vi "Write Values and Check for Stabilization.vi"(0 "DataCluster In":T1, 5 "DesiredParameters":T3={"Para1"=0, "SP1"=0.0, "Para2"=1, "SP2"=0.0, "Para3"=4, "SP3"=10.0}, 7 "Stability Cluster":T2, 9 "Controller?":bool, 11 "DataDisplayRefs":refnum<vi>[](array[refnum]), 13 "StabilizedRef":refnum<vi>) -> (4 "DataCluster Out":T1)   [LabVIEW 2019]
uses:
  TypeDef/DataCluster.ctl
  TypeDef/Command Cluster.ctl
  TypeDef/Stability Cluster.ctl
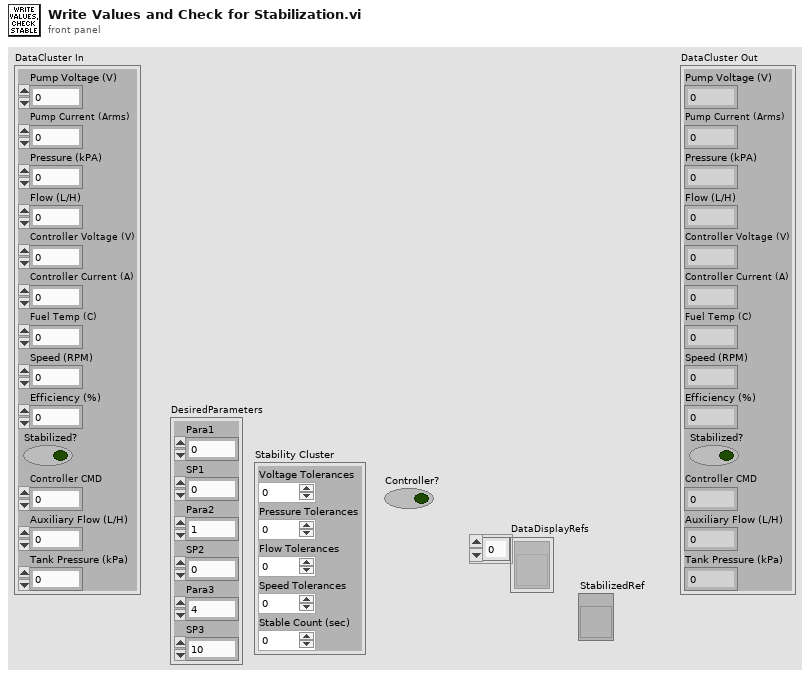
[diagram p1: front panel]
types:
  T1 = typedef "DataCluster.ctl" = cluster{"Pump Voltage (V)":dbl, "Pump Current (Arms)":dbl, "Pressure (kPA)":dbl, "Flow (L/H)":dbl, "Controller Voltage (V)":dbl, "Controller Current (A)":dbl, "Fuel Temp (C)":dbl, "Speed (RPM)":dbl, "Efficiency (%)":dbl, "Stabilized?":bool, "Controller CMD":dbl, "Auxiliary Flow (L/H)":dbl, "Tank Pressure (kPa)":dbl}
  T2 = typedef "Stability Cluster.ctl" = cluster{"Voltage Tolerances":dbl, "Pressure Tolerances":dbl, "Flow Tolerances":dbl, "Speed Tolerances":dbl, "Stable Count (sec)":dbl}
  T3 = typedef "Command Cluster.ctl" = cluster{"Para1":i32, "SP1":dbl, "Para2":i32, "SP2":dbl, "Para3":i32, "SP3":dbl}
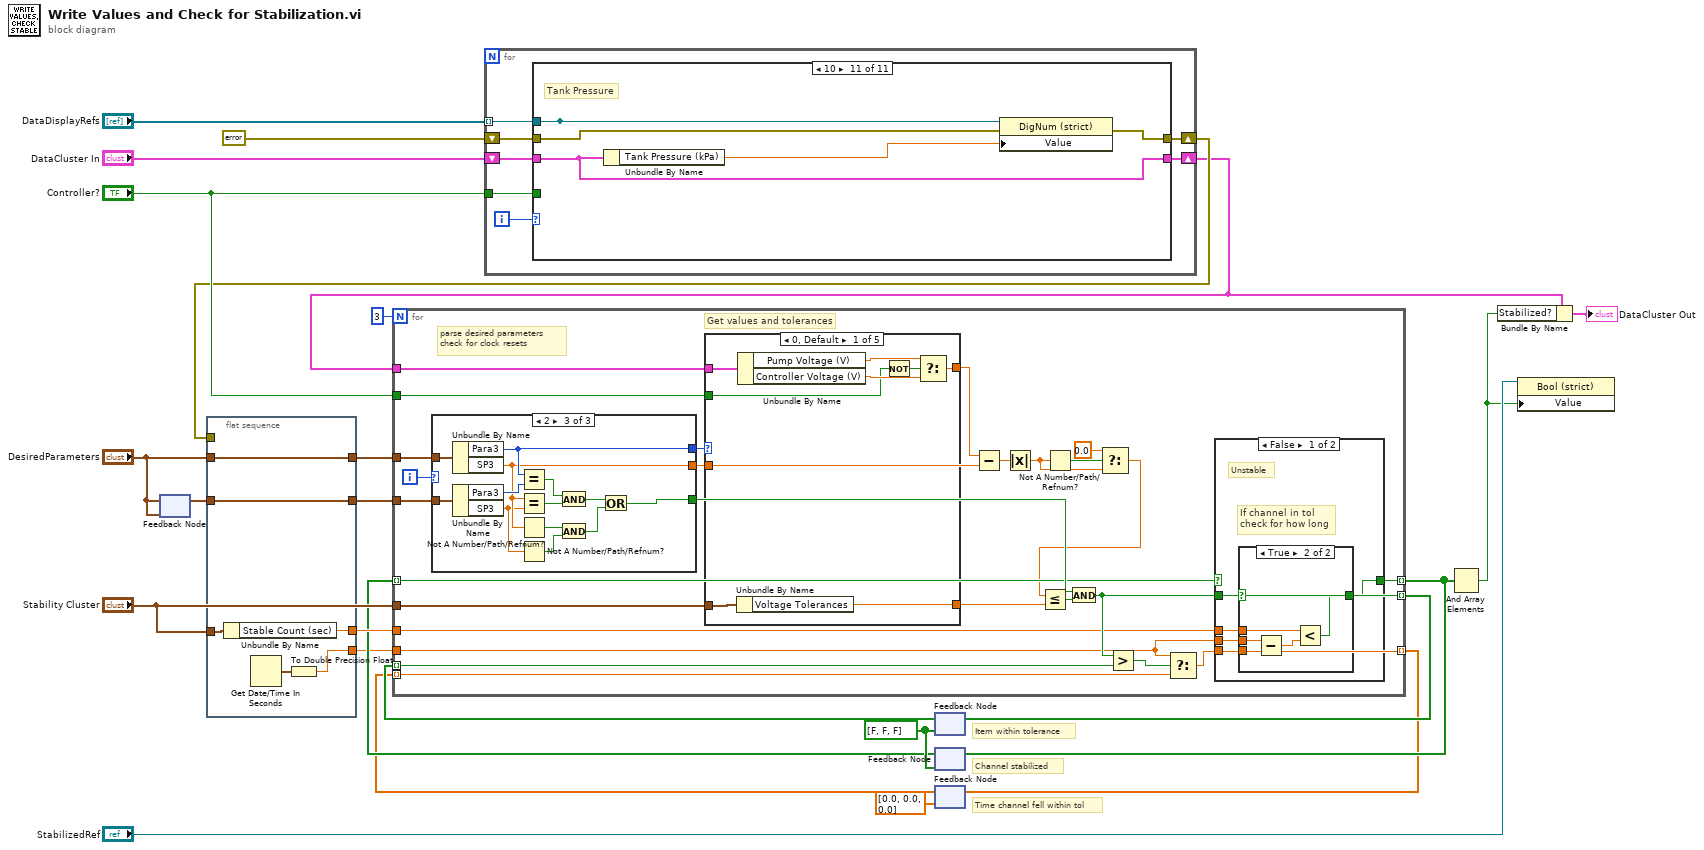
[diagram p0: block diagram]
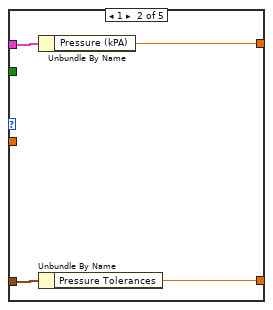
[diagram p4: hidden frame]
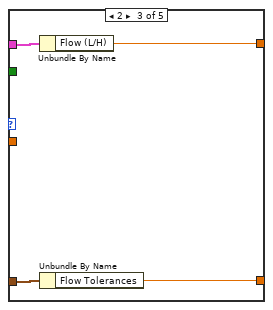
[diagram p5: hidden frame]
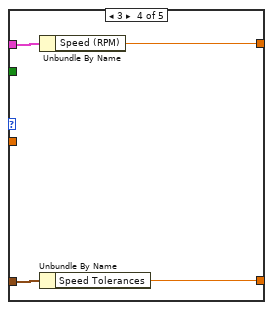
[diagram p6: hidden frame]
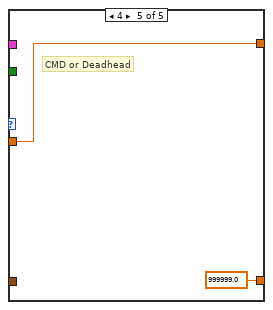
[diagram p7: hidden frame]
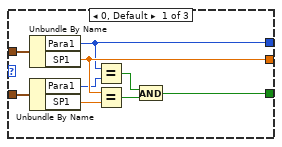
[diagram p8: hidden frame]
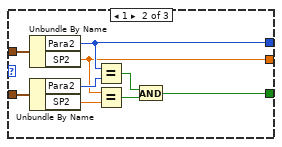
[diagram p9: hidden frame]
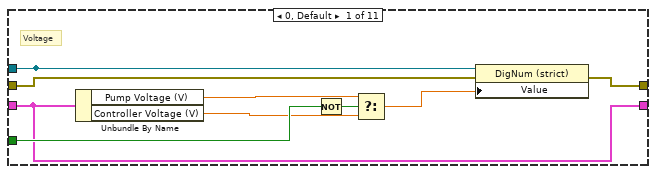
[diagram p10: hidden frame]
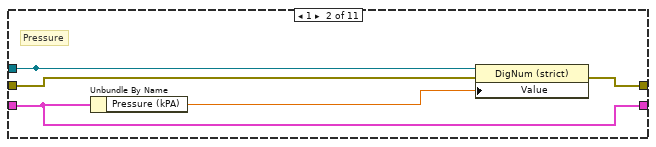
[diagram p11: hidden frame]
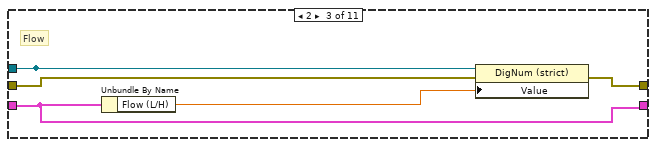
[diagram p12: hidden frame]
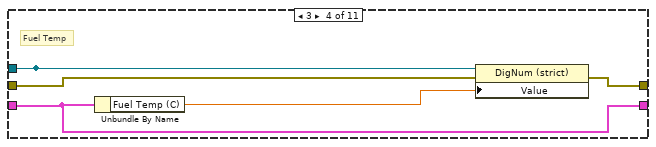
[diagram p13: hidden frame]
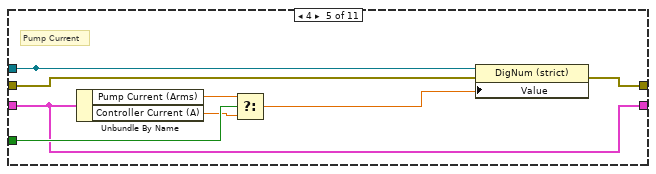
[diagram p14: hidden frame]
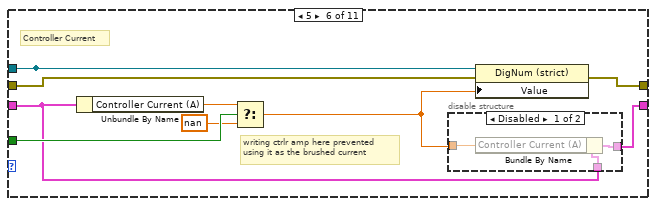
[diagram p15: hidden frame]
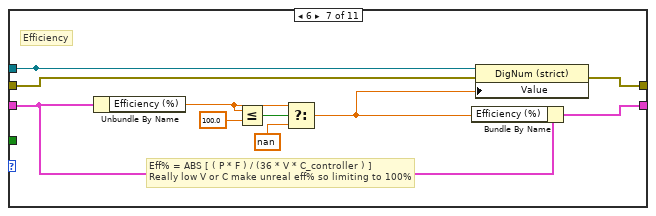
[diagram p17: hidden frame]
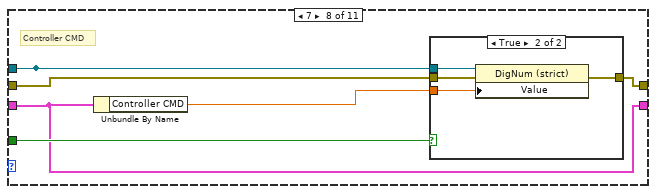
[diagram p18: hidden frame]
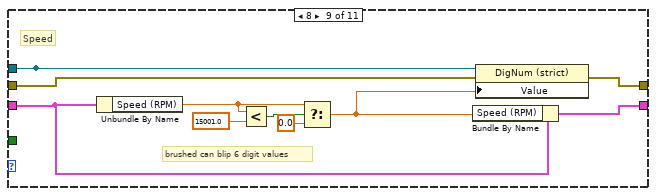
[diagram p20: hidden frame]
diagram:
  w18 = bool[] [FALSE, FALSE, FALSE]
  # "Time channel fell within tol"
  # "Channel stabilized"
  # "Item within tolerance"
  n1 = feedback-in #1("DesiredParameters") -> ()
  n2 = feedback #1("DesiredParameters") -> (w7:T3)
  n3 = flat-sequence {
    tunnel: "Stability Cluster" -> [w31]
    tunnel: [w30] -> w21
    tunnel: "DesiredParameters" -> [w29]
    tunnel: w7 -> [w28]
    tunnel: [w29] -> w6
    tunnel: [w28] -> w5
    tunnel: [w26] -> w4
    tunnel: w3 -> [_]
    frame #0 {
      n4 = Unbundle By Name(w31) -> ("Stable Count (sec)"=w30:dbl)
      n5 = Get Date/Time In Seconds() -> (seconds since 1Jan1904=w27:timestamp)
      n6 = To Double Precision Float(number=w27) -> (double precision float=w26:dbl)
    }
  }
  n7 = for {
    tunnel: "Controller?" -> [w36]
    tunnel: "DataDisplayRefs" -> [w35] mode=indexing
    shift-right: [w33] -> w3
    shift-left: errorcluster {"status"=FALSE, "code"=0, "source"=""} ("error in (no error)") -> [w34]
    shift-right: [w32] -> w1
    shift-left: "DataCluster In" -> [w37]
    i -> [w38]
    n8 = case shown="10" w38 {
      tunnel: w37 -> [w39 w48 w53 w58 w63 w73 w86 w94 w107 w115 w120]
      tunnel: w36 -> [w46 _ _ _ w67 w77 _ w97 _ _ _]
      tunnel: [w43 w52 w57 w62 w70 w79 w93 w99 w114 w119 w124] -> _
      tunnel: w35 -> [w43 w52 w57 w62 w70 w79 w93 w99 w114 w119 w124]
      tunnel: w34 -> [w41 w49 w55 w60 w65 w75 w88 w96 w109 w118 w123]
      tunnel: [w40 w50 w54 w59 w64 w74 w87 w95 w108 w117 w122] -> w33
      tunnel: [w39 w48 w53 w58 w63 w71 w85 w94 w105 w115 w120] -> w32
      frame 0, Default {
        # "Voltage"
        n9 = Unbundle By Name(w39) -> ("Pump Voltage (V)"=w45:dbl, "Controller Voltage (V)"=w44:dbl)
        n10 = Not(x=w46) -> (.not. x?=w47:bool)
        n11 = Select(t=w45, s=w47, f=w44) -> (s? t:f=w42:dbl)
        n12 = property class="DigNum (strict)"(reference=w43, error in=w41, "Value"=w42) -> (error out=w40:errorcluster)  [unwired: 1 out]
      }
      frame 1 {
        # "Pressure"
        n13 = Unbundle By Name(w48) -> ("Pressure (kPA)"=w51:dbl)
        n14 = property class="DigNum (strict)"(reference=w52, error in=w49, "Value"=w51) -> (error out=w50:errorcluster)  [unwired: 1 out]
      }
      frame 2 {
        # "Flow"
        n15 = Unbundle By Name(w53) -> ("Flow (L/H)"=w56:dbl)
        n16 = property class="DigNum (strict)"(reference=w57, error in=w55, "Value"=w56) -> (error out=w54:errorcluster)  [unwired: 1 out]
      }
      frame 3 {
        # "Fuel Temp"
        n17 = Unbundle By Name(w58) -> ("Fuel Temp (C)"=w61:dbl)
        n18 = property class="DigNum (strict)"(reference=w62, error in=w60, "Value"=w61) -> (error out=w59:errorcluster)  [unwired: 1 out]
      }
      frame 4 {
        # "Pump Current"
        n19 = Unbundle By Name(w63) -> ("Pump Current (Arms)"=w69:dbl, "Controller Current (A)"=w66:dbl)
        n20 = Select(t=w69, s=w67, f=w66) -> (s? t:f=w68:dbl)
        n21 = property class="DigNum (strict)"(reference=w70, error in=w65, "Value"=w68) -> (error out=w64:errorcluster)  [unwired: 1 out]
      }
      frame 5 {
        # "writing ctrlr amp here prevented\nusing it as the brushed current"
        # "Controller Current"
        n22 = Unbundle By Name(w73) -> ("Controller Current (A)"=w78:dbl)
        n23 = Select(t=w78, s=w77, f=nan) -> (s? t:f=w72:dbl)
        n24 = disable-structure shown="Disabled" {
          disable-tunnel: w73 -> [w82 w83]
          disable-tunnel: w72 -> [w81 _]
          disable-tunnel: [w80 w83] -> w71
          frame Disabled {
            n25 = Bundle By Name(cluster=w82, "Controller Current (A)"=w81) -> (w80:T1)
          }
          frame Enabled {
          }
        }
        n26 = property class="DigNum (strict)"(reference=w79, error in=w75, "Value"=w72) -> (error out=w74:errorcluster)  [unwired: 1 out]
      }
      frame 6 {
        # "Eff% = ABS [ ( P * F ) / (36 * V * C_controller ) ]\nReally low V or C make unreal eff% so limiting to 100%"
        # "Efficiency"
        n27 = Unbundle By Name(w86) -> ("Efficiency (%)"=w89:dbl)
        n28 = Less Or Equal?(x=w89, y=100.0) -> (x <= y?=w92:bool)
        n29 = Select(t=w89, s=w92, f=nan) -> (s? t:f=w84:dbl)
        n30 = Bundle By Name(cluster=w86, "Efficiency (%)"=w84) -> (w85:T1)
        n31 = property class="DigNum (strict)"(reference=w93, error in=w88, "Value"=w84) -> (error out=w87:errorcluster)  [unwired: 1 out]
      }
      frame 7 {
        # "Controller CMD"
        n32 = Unbundle By Name(w94) -> ("Controller CMD"=w98:dbl)
        n33 = case shown="True" w97 {
          tunnel: w99 -> [_ w104]
          tunnel: w98 -> [_ w103]
          tunnel: w96 -> [w100 w102]
          tunnel: [w100 w101] -> w95
          frame False {
          }
          frame True {
            n34 = property class="DigNum (strict)"(reference=w104, error in=w102, "Value"=w103) -> (error out=w101:errorcluster)  [unwired: 1 out]
          }
        }
      }
      frame 8 {
        # "brushed can blip 6 digit values"
        # "Speed"
        n35 = Unbundle By Name(w107) -> ("Speed (RPM)"=w110:dbl)
        n36 = Less?(x=w110, y=15001.0) -> (x < y?=w111:bool)
        n37 = Select(t=w110, s=w111, f=0.0) -> (s? t:f=w106:dbl)
        n38 = Bundle By Name(cluster=w107, "Speed (RPM)"=w106) -> (w105:T1)
        n39 = property class="DigNum (strict)"(reference=w114, error in=w109, "Value"=w106) -> (error out=w108:errorcluster)  [unwired: 1 out]
      }
      frame 9 {
        # "Auxiliary Flow"
        n40 = Unbundle By Name(w115) -> ("Auxiliary Flow (L/H)"=w116:dbl)
        n41 = property class="DigNum (strict)"(reference=w119, error in=w118, "Value"=w116) -> (error out=w117:errorcluster)  [unwired: 1 out]
      }
      frame 10 {
        # "Tank Pressure"
        n42 = Unbundle By Name(w120) -> ("Tank Pressure (kPa)"=w121:dbl)
        n43 = property class="DigNum (strict)"(reference=w124, error in=w123, "Value"=w121) -> (error out=w122:errorcluster)  [unwired: 1 out]
      }
    }
  }
  n44 = feedback #2(w18) -> (w19:bool[])
  n45 = feedback #3(w18) -> (w17:bool[])
  n46 = feedback #4(dbl[] [0.0, 0.0, 0.0]) -> (w12:dbl[])
  n47 = for {
    N: 3 -> [_]
    tunnel: w6 -> [w149]
    tunnel: w1 -> [w147]
    tunnel: "Controller?" -> [w146]
    tunnel: "Stability Cluster" -> [w142]
    tunnel: w21 -> [w129]
    tunnel: w5 -> [w141]
    tunnel: [w135] -> w20 mode=indexing
    tunnel: w19 -> [w137] mode=indexing
    tunnel: [w134] -> w16 mode=indexing
    tunnel: w17 -> [w136] mode=indexing
    tunnel: w12 -> [w132] mode=indexing
    tunnel: [w130] -> w14 mode=indexing
    tunnel: w4 -> [w131]
    i -> [w150]
    # "Get values and tolerances"
    # "parse desired parameters\ncheck for clock resets"
    n48 = case shown="2" w150 {
      tunnel: w149 -> [w193 w202 w215]
      tunnel: [w186 w197 w212] -> w148
      tunnel: [w187 w196 w206] -> w145
      tunnel: w141 -> [w192 w201 w214]
      tunnel: [w189 w194 w203] -> w138
      frame 0, Default {
        n49 = Unbundle By Name(w193) -> ("Para1"=w186:i32, "SP1"=w187:dbl)
        n50 = Unbundle By Name(w192) -> ("Para1"=w185:i32, "SP1"=w188:dbl)
        n51 = Equal?(x=w186, y=w185) -> (x = y?=w190:bool)
        n52 = Equal?(x=w187, y=w188) -> (x = y?=w191:bool)
        n53 = And(x=w190, y=w191) -> (x .and. y?=w189:bool)
      }
      frame 1 {
        n54 = Unbundle By Name(w202) -> ("Para2"=w197:i32, "SP2"=w196:dbl)
        n55 = Unbundle By Name(w201) -> ("Para2"=w198:i32, "SP2"=w195:dbl)
        n56 = Equal?(x=w197, y=w198) -> (x = y?=w199:bool)
        n57 = Equal?(x=w196, y=w195) -> (x = y?=w200:bool)
        n58 = And(x=w199, y=w200) -> (x .and. y?=w194:bool)
      }
      frame 2 {
        n59 = Unbundle By Name(w215) -> ("Para3"=w212:i32, "SP3"=w206:dbl)
        n60 = Unbundle By Name(w214) -> ("Para3"=w213:i32, "SP3"=w205:dbl)
        n61 = Equal?(x=w212, y=w213) -> (x = y?=w210:bool)
        n62 = Equal?(x=w206, y=w205) -> (x = y?=w211:bool)
        n63 = Not A Number/Path/Refnum?(number/path/refnum=w206) -> (NaN/Path/Refnum?=w209:bool)
        n64 = Not A Number/Path/Refnum?(number/path/refnum=w205) -> (NaN/Path/Refnum?=w208:bool)
        n65 = And(x=w210, y=w211) -> (x .and. y?=w204:bool)
        n66 = And(x=w209, y=w208) -> (x .and. y?=w207:bool)
        n67 = Or(x=w204, y=w207) -> (x .or. y?=w203:bool)
      }
    }
    n68 = case shown="0, Default" w148 {
      tunnel: w147 -> [w167 w174 w178 w182 _]
      tunnel: w146 -> [w166 _ _ _ _]
      tunnel: [w165 w173 w177 w181 w184] -> w144
      tunnel: w145 -> [_ _ _ _ w184]
      tunnel: w142 -> [w164 w172 w176 w180 _]
      tunnel: [w163 w171 w175 w179 999999.0 ("Speed Tolerances")] -> w140
      frame 0, Default {
        n69 = Unbundle By Name(w164) -> ("Voltage Tolerances"=w163:dbl)
        n70 = Unbundle By Name(w167) -> ("Pump Voltage (V)"=w169:dbl, "Controller Voltage (V)"=w170:dbl)
        n71 = Not(x=w166) -> (.not. x?=w168:bool)
        n72 = Select(t=w169, s=w168, f=w170) -> (s? t:f=w165:dbl)
      }
      frame 1 {
        n73 = Unbundle By Name(w174) -> ("Pressure (kPA)"=w173:dbl)
        n74 = Unbundle By Name(w172) -> ("Pressure Tolerances"=w171:dbl)
      }
      frame 2 {
        n75 = Unbundle By Name(w178) -> ("Flow (L/H)"=w177:dbl)
        n76 = Unbundle By Name(w176) -> ("Flow Tolerances"=w175:dbl)
      }
      frame 3 {
        n77 = Unbundle By Name(w182) -> ("Speed (RPM)"=w181:dbl)
        n78 = Unbundle By Name(w180) -> ("Speed Tolerances"=w179:dbl)
      }
      frame 4 {
        # "CMD or Deadhead"
      }
    }
    n79 = Subtract(x=w144, y=w145) -> (x-y=w143:dbl)
    n80 = Absolute Value(x=w143) -> (abs(x)=w126:dbl)
    n81 = Not A Number/Path/Refnum?(number/path/refnum=w126) -> (NaN/Path/Refnum?=w128:bool)
    n82 = Select(t=0.0, s=w128, f=w126) -> (s? t:f=w125:dbl)
    n83 = Less Or Equal?(x=w125, y=w140) -> (x <= y?=w139:bool)
    n84 = And(x=w138, y=w139) -> (x .and. y?=w135:bool)
    n85 = Greater?(x=w135, y=w137) -> (0:w133:bool)
    n86 = Select(t=w131, s=w133, f=w132) -> (s? t:f=w130:dbl)
    n87 = case shown="False" w136 {
      tunnel: w135 -> [w153 w162]
      tunnel: [w152 w162] -> w134
      tunnel: w131 -> [w155 _]
      tunnel: w130 -> [w154 _]
      tunnel: w129 -> [w151 _]
      frame False {
        # "If channel in tol\ncheck for how long"
        # "Unstable"
        n88 = case shown="True" w153 {
          selector: w153 -> [w156 _]
          tunnel: w155 -> [_ w161]
          tunnel: w154 -> [_ w160]
          tunnel: [w156 w157] -> w152
          tunnel: w151 -> [_ w159]
          frame False {
          }
          frame True {
            n89 = Subtract(x=w161, y=w160) -> (x-y=w158:dbl)
            n90 = Less?(x=w159, y=w158) -> (x < y?=w157:bool)
          }
        }
      }
      frame True {
        # "Stable\nlook to kick"
      }
    }
  }
  n91 = feedback-in #2(w20) -> ()
  n92 = feedback-in #3(w16) -> ()
  n93 = feedback-in #4(w14) -> ()
  n94 = And Array Elements(Boolean array=w16) -> (logical AND=w10:bool)
  n95 = Bundle By Name(cluster=w1, "Stabilized?"=w10) -> (→"DataCluster Out":T1)
  n96 = property class="Bool (strict)"(reference="StabilizedRef", "Value"=w10) -> ()  [unwired: 1 in, 2 out]
